vi "Write Configuration.vi"(8 "error in (no error)":errorcluster, 10 "Configuration":T1, 11 "RandomNumberLogger in":refnum<class "RandomNumberLogger.lvclass">) -> (0 "error out":errorcluster, 2 "Configure and Synchronize Required":bool, 3 "RandomNumberLogger out":refnum<class "RandomNumberLogger.lvclass">)   [LabVIEW 2020, in "RandomNumberLogger.lvlib" / "RandomNumberLogger.lvclass"]
doc: "<b>Write Configuration</b>\nBy default just store specified configuration and signal the PE state machine to reconfigure the PE"
uses:
  RandomNumberLogger.lvclass
  RandomNumberLogger.lvclass/RandomNumberLogger.ctl
  Configuration.ctl
panel:
  # "#via_ignore"
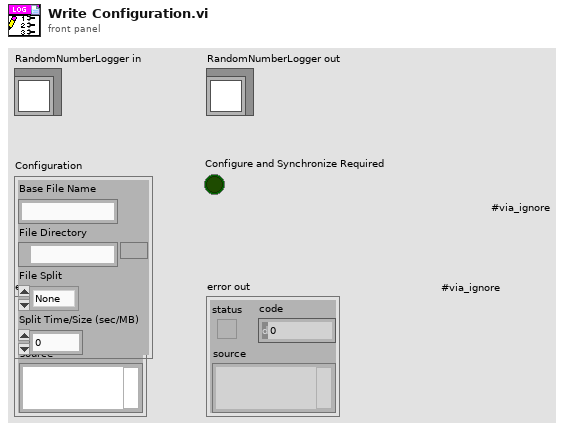
[diagram p1: front panel]
types:
  T1 = typedef "RandomNumberLogger.lvlib/RandomNumberLogger.lvclass/Configuration.ctl" = cluster{"Base File Name":string, "File Directory":path, "File Split":enum16{"None", "Time", "Size"}, "Split Time/Size (sec/MB)":dbl}
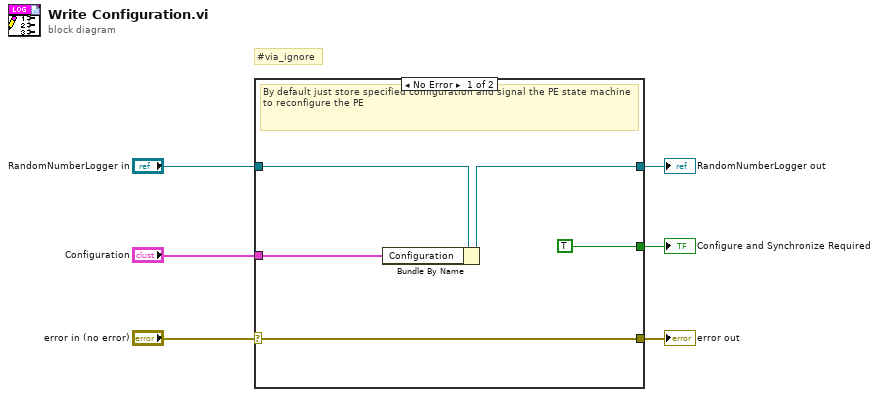
[diagram p0: block diagram]
diagram:
  # "#via_ignore"
  n1 = case shown="No Error" "error in (no error)" {
    selector: "error in (no error)" -> [w11 w12]
    tunnel: [w11 w12] -> w5
    tunnel: [w9 w13] -> w3
    tunnel: "RandomNumberLogger in" -> [w10 w13]
    tunnel: "Configuration" -> [w8 _]
    tunnel: [TRUE ("Configure and Synchronize Required") _] -> w1
    frame No Error {
      # "By default just store specified configuration and signal the PE state machine to reconfigure the PE"
      n2 = Bundle By Name(cluster=w10, "Configuration"=w8) -> (w9:refnum<class "RandomNumberLogger.lvclass">)
    }
    frame Error {
    }
  }
  "error out" <- w5
  "RandomNumberLogger out" <- w3
  "Configure and Synchronize Required" <- w1
